vi "GetExternalInterfaces.vi"(8 "ErrorIn":errorcluster, 11 "ReferenceIn":refnum<class "TAFBaseGUI.lvclass">) -> (0 "ErrorOut":errorcluster, 2 "ExternalInterfaces":T1[](array[typedef]), 3 "ReferenceOut":refnum<class "TAFBaseGUI.lvclass">)   [LabVIEW 2021, in "TAFBaseGUI.lvclass"]
uses:
  TAFBaseGUI.lvclass
  Library_TAF_Support/ClusterArrayConversion/BundledArray.ctl
  Library_TAF_Support/ClusterArrayConversion/ClusterArrayConversion.lvlib
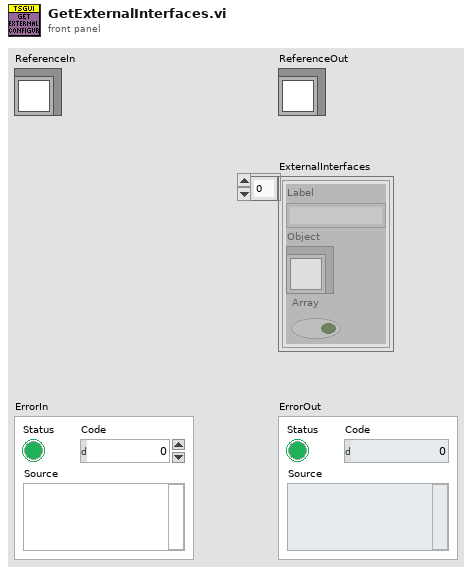
[diagram p1: front panel]
types:
  T1 = typedef "ClusterArrayConversion.lvlib/BundledArray.ctl" = cluster{"Label":string, "Object":refnum<class>, "Array":bool}
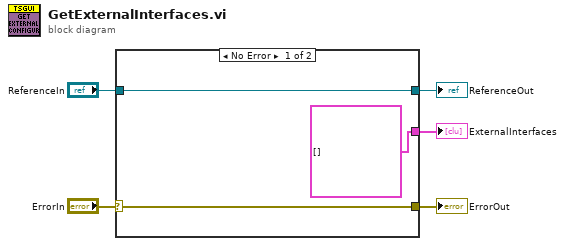
[diagram p0: block diagram]
diagram:
  n1 = case shown="No Error" "ErrorIn" {
    selector: "ErrorIn" -> [w8 w10]
    tunnel: [w8 w10] -> w4
    tunnel: [w7 w9] -> w2
    tunnel: "ReferenceIn" -> [w7 w9]
    tunnel: [T1[] [] ("BundeledLabels") _] -> w1
    frame No Error {
    }
    frame Error {
    }
  }
  "ErrorOut" <- w4
  "ReferenceOut" <- w2
  "ExternalInterfaces" <- w1
